vi "numerospares.vi"() -> ()   [LabVIEW 2011]
panel:
  out "Array":dbl[](array[numeric])
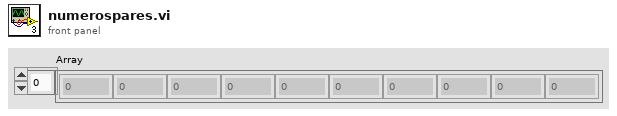
[diagram p1: front panel]
types:
  T1 = enum16{"open", "replace", "create", "open or create", "replace or create", "replace or create with confirmation"}
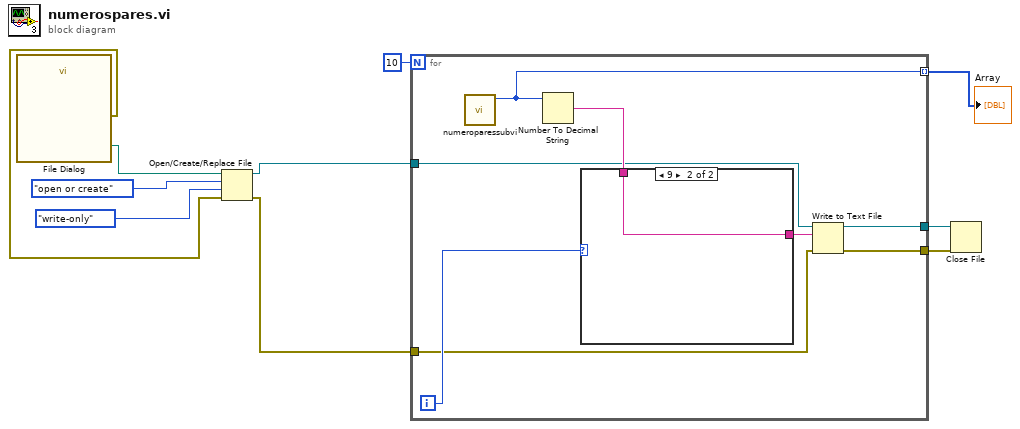
[diagram p0: block diagram]
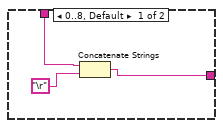
[diagram p2: hidden frame]
diagram:
  n1 = call "File Dialog"() -> ("selected path"=w10:path, "error out"=w9:errorcluster)  [unwired: 12 in, 2 out]
  n2 = Open/Create/Replace File(file path (use dialog)=w10, error in=w9, operation (0:open)=T1."open or create", access (0:read/write)=enum16{"read/write", "read-only", "write-only"}."write-only") -> (refnum out=w4:refnum<file>, error out=w5:errorcluster)  [unwired: 2 in, 1 out]
  n3 = for {
    N: 10 -> [_]
    tunnel: w5 -> [w15]
    tunnel: w4 -> [w14]
    tunnel: [w13] -> w3
    tunnel: [w12] -> w2
    tunnel: [w11] -> w1 mode=indexing
    i -> [w18]
    n4 = call "numeroparessubvi.vi"() -> ("Numeric"=w11:i32)  [unwired: 11 in]
    n5 = Number To Decimal String(number=w11) -> (decimal integer string=w17:string)  [unwired: 1 in]
    n6 = case shown="9" w18 {
      tunnel: w17 -> [w21 w22]
      tunnel: [w19 w22] -> w16
      frame 0..8, Default {
        n7 = Concatenate Strings "Concatenate Strings"(w21, "\r") -> (w19:string)
      }
      frame 9 {
      }
    }
    n8 = Write to Text File(file (use dialog)=w14, text=w16, error in=w15) -> (refnum out=w13:refnum<file>, error out=w12:errorcluster)  [unwired: 1 in, 1 out]
  }
  "Array" <- w1
  n9 = Close File(refnum=w3, error in=w2) -> ()  [unwired: 2 out]
